vi "Test_AO.vi"() -> ()   [LabVIEW 2023]
uses:
  Driver_AI_AO/Driver_AI_AO.lvclass
panel:
  in  "PWM":u8
  in  "Input":T1
  out "STATUS":string
  out "error out":errorcluster
  out "Error":string
  in  "PIN":i8
  in  "error in (no error)":errorcluster
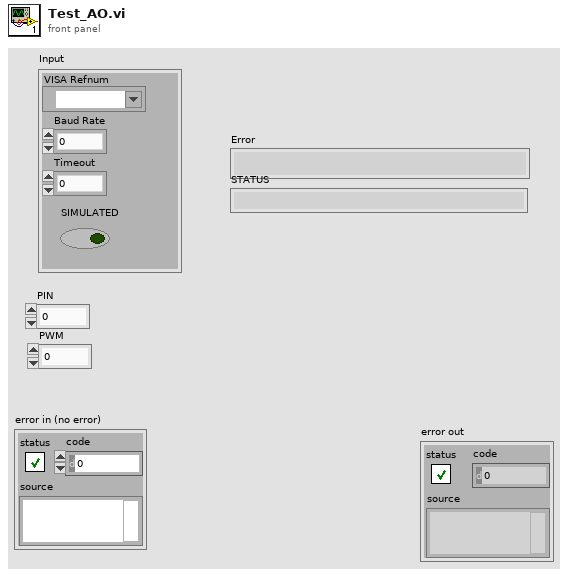
[diagram p1: front panel]
types:
  T1 = cluster{"VISA Refnum":refnum<visa-resource-name>, "Baud Rate":u32, "Timeout":u32, "SIMULATED":bool}
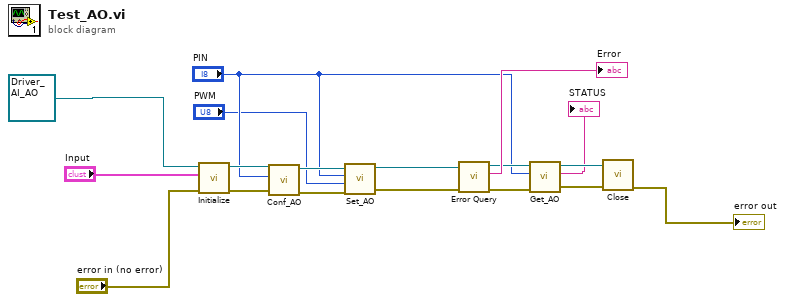
[diagram p0: block diagram]
diagram:
  n1 = call-dynamic "Initialize.vi"("error in (no error)"="error in (no error)", "Input"="Input", "Driver in"=refnum<class "Driver_AI_AO.lvclass"> refnum ("Driver_AI_AO.lvlib:Driver_AI_AO.lvclass")) -> ("error out"=w12:errorcluster, "Driver out"=w13:refnum<class "Driver_AI_AO.lvclass">)  [unwired: 7 in]
  n2 = call-dynamic "Conf_AO.vi"("error in (no error)"=w12, "PIN Number"="PIN", "Driver_AI_AO in"=w13) -> ("error out"=w11:errorcluster, "Driver_AI_AO out"=w10:refnum<class "Driver_AI_AO.lvclass">)  [unwired: 7 in]
  n3 = call-dynamic "Set_AO.vi"("error in (no error)"=w11, "PWM"="PWM", "PIN"="PIN", "Driver_AI_AO in"=w10) -> ("error out"=w9:errorcluster, "Driver_AI_AO out"=w8:refnum<class "Driver_AI_AO.lvclass">)  [unwired: 6 in]
  n4 = call-dynamic "Error Query.vi"("error in (no error)"=w9, "Driver in"=w8) -> ("error out"=w7:errorcluster, "read buffer"=→"Error":string, "Driver out"=w3:refnum<class "Driver_AI_AO.lvclass">)  [unwired: 7 in]
  n5 = call-dynamic "Get_AO.vi"("error in (no error)"=w7, "PIN Number"="PIN", "Driver_AI_AO in"=w3) -> ("error out"=w6:errorcluster, "STATUS"=→"STATUS":string, "Driver_AI_AO out"=w5:refnum<class "Driver_AI_AO.lvclass">)  [unwired: 6 in]
  n6 = call-dynamic "Close.vi"("error in (no error)"=w6, "Driver in"=w5) -> ("error out"=→"error out":errorcluster)  [unwired: 8 in, 1 out]
